vi "Make JSON Array.vi"(6 "Pretty Print?":bool, 8 "error in (no error)":errorcluster, 9 "JSON Elements":string[](array[string])) -> (0 "error out":errorcluster, 3 "<JSON>":string caption="<JSON>Array")   [LabVIEW 2020, in "JSONtext.lvlib"]
doc: "Format a JSON Array out of an array of JSON items."
uses:
  <vilib>/JDP Science/JSONtext/JSONtext.lvlib
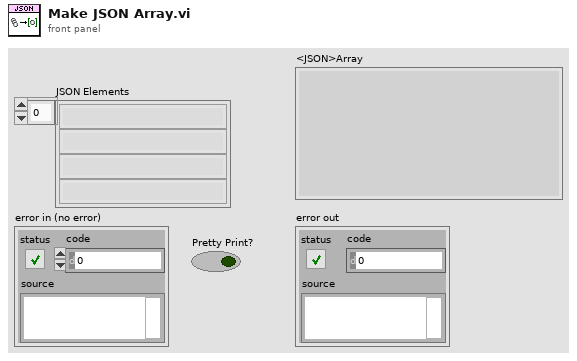
[diagram p1: front panel]
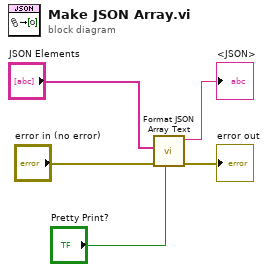
[diagram p0: block diagram]
diagram:
  n1 = call <vilib>:"Format JSON Array Text.vi"("Pretty Print?"="Pretty Print?", "error in (no error)"="error in (no error)", "Array of JSON Text"="JSON Elements") -> ("error out"=→"error out":errorcluster, "<JSON>"=→"<JSON>":string)  [unwired: 7 in]
